vi "Add Chassis Dialog.vi"(8 "error in (no error)":errorcluster, 11 "hostname":string) -> (0 "error out":errorcluster, 2 "Result":T1, 3 "Cancelled?":bool)   [LabVIEW 2017]
doc: "Use this template to create a dialog box with event handling."
panel:
  in  "password":string
  in  "username":string="admin"
  in  "Cancel":bool
  in  "OK":bool
  # "Hostname or IP Address"
  # "Username"
  # "Password"
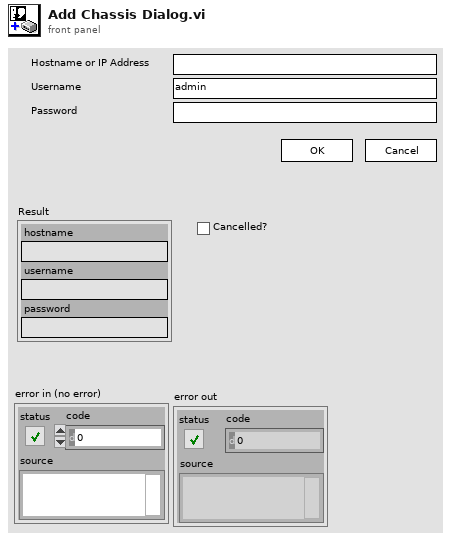
[diagram p1: front panel]
types:
  T1 = cluster{"hostname":string, "username":string, "password":string}
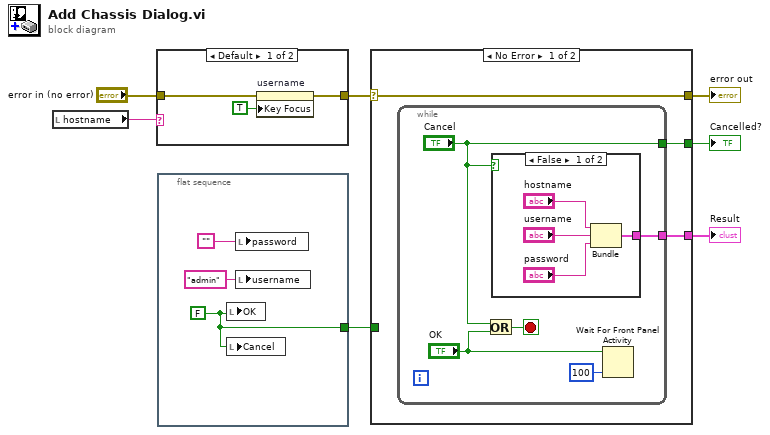
[diagram p0: block diagram]
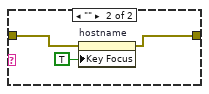
[diagram p2: hidden frame]
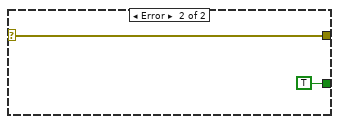
[diagram p4: hidden frame]
diagram:
  n1 = local read "hostname"() -> (w1:string)
  n2 = case shown="Default" w1 {
    tunnel: "error in (no error)" -> [w9 w12]
    tunnel: [w8 w11] -> w2
    frame Default {
      n3 = property on="username" class="Str"(error in=w9, "Key Focus"=TRUE) -> (error out=w8:errorcluster)  [unwired: 1 in, 1 out]
    }
    frame "" {
      n4 = property on="hostname" class="Str"(error in=w12, "Key Focus"=TRUE) -> (error out=w11:errorcluster)  [unwired: 1 in, 1 out]
    }
  }
  n5 = flat-sequence {
    tunnel: [w15] -> w4
    frame #0 {
      w15 = FALSE
      n6 = local write "OK"(w15) -> ()
      n7 = local write "Cancel"(w15) -> ()
      n8 = local write "password"("") -> ()
      n9 = local write "username"("admin" ("username")) -> ()
    }
  }
  n10 = case shown="No Error" w2 {
    selector: w2 -> [w19 w30]
    tunnel: [w19 w30] -> w7
    tunnel: [w17 TRUE] -> w5
    tunnel: [w18 _] -> w6
    tunnel: w4 -> [_ _]
    frame No Error {
      n11 = while {
        tunnel: [w24] -> w18
        tunnel: ["Cancel"] -> w17
        stop <- w22 stop-if-true
        n12 = Or(x="Cancel", y="OK") -> (x .or. y?=w22:bool)
        n13 = case shown="False" "Cancel" {
          tunnel: [w25 _] -> w24
          frame False {
            n14 = Bundle("hostname"="hostname", "username"="username", "password"="password") -> (w25:T1)  [unwired: 1 in]
          }
          frame True {
          }
        }
        n15 = Wait For Front Panel Activity(1:100 ("timeout ms (-1 never timeout)"), 3:"OK") -> ()  [unwired: 1 in, 1 out]
      }
    }
    frame Error {
    }
  }
  "Cancelled?" <- w5
  "Result" <- w6
  "error out" <- w7
